vi "RetrieveImage_Main.vi"(8 "error in (no error)":errorcluster, 11 "DevInfo":T1={"Hostname"="", "IPAddress"="", "MAC"="", "SerialNum"="", "Model"="", "Status"="", "FW"="", "OSDesc"="", "ImgTitle"="", "ImgDesc"="", "ImgVer"="", "ImgID"="", "IP Address Request Mode"=1, "SubnetMask"="", "Gateway"="", "DNSServer"=""} {"IP Address Request Mode" items=["Static"=1, "DHCP/Link-Local"=2, "Link-Local Only"=4, "DHCP Only"=8]}) -> (0 "error out":errorcluster)   [LabVIEW 2021]
uses:
  TypeDefs/DevInfo.ctl
  TypeDefs/RetrieveImageStates.ctl
  TypeDefs/AppImageProperties.ctl
  TypeDefs/FPGA_Properties_Element.ctl
  <vilib>/nisyscfg/Software 1.2.ctl
  <vilib>/nisyscfg/Component Type.ctl
  <vilib>/nisyscfg/nisyscfg.lvlib
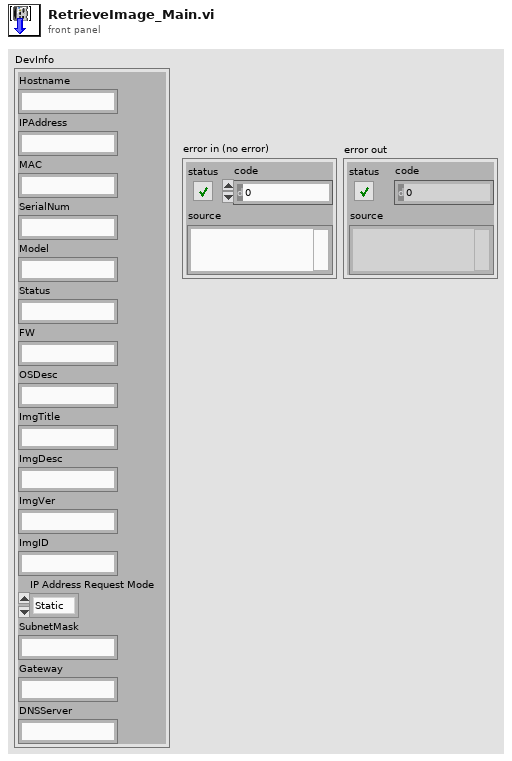
[diagram p1: front panel]
types:
  T1 = typedef "DevInfo.ctl" = cluster{"Hostname":string, "IPAddress":string, "MAC":string, "SerialNum":string, "Model":string, "Status":string, "FW":string, "OSDesc":string, "ImgTitle":string, "ImgDesc":string, "ImgVer":string, "ImgID":string, "IP Address Request Mode":i32, "SubnetMask":string, "Gateway":string, "DNSServer":string}
  T2 = typedef "AppImageProperties.ctl" = cluster{"Name":string, "Version":string, "Time":timestamp, "Description":string, "Key":string, "Chassis":string, "FPGA Properties":T3[], "Model":string, "Retrieve":string[], "Deploy":string[], "Installed Software":string[]}
  T3 = typedef "FPGA_Properties_Element.ctl" = cluster{"Resource Name":string, "Path":path}
  T4 = typedef "RetrieveImageStates.ctl" = enum16{"Get Target Image Info", "Set Image Properties", "Get Installed Software", "Retrieve Image", "Package Image", "Clean Up", "Exit"}
  T5 = cluster{"AppImage Properties":T2, "Image Filepath":path}
  T6 = typedef "nisyscfg.lvlib/Software 1.2.ctl" = cluster{"title":string, "description":string, "ID":string, "version":string, "component type":T7}
  T7 = typedef "nisyscfg.lvlib/Component Type.ctl" = u32
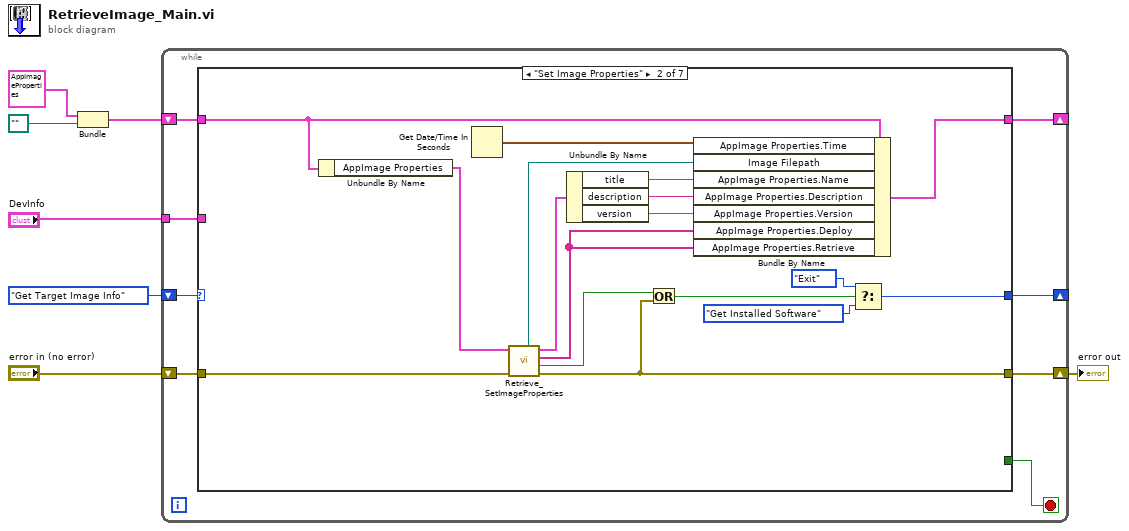
[diagram p0: block diagram]
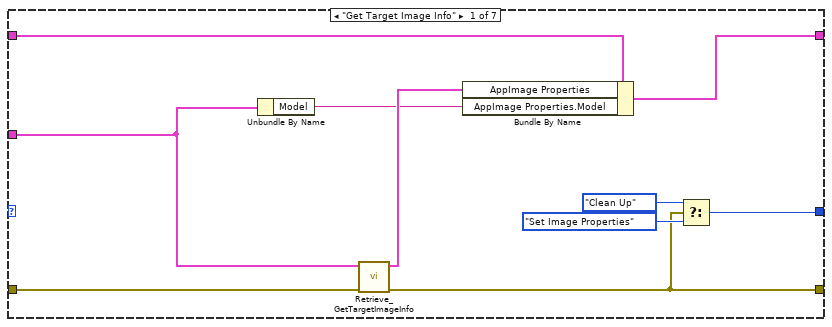
[diagram p2: hidden frame]
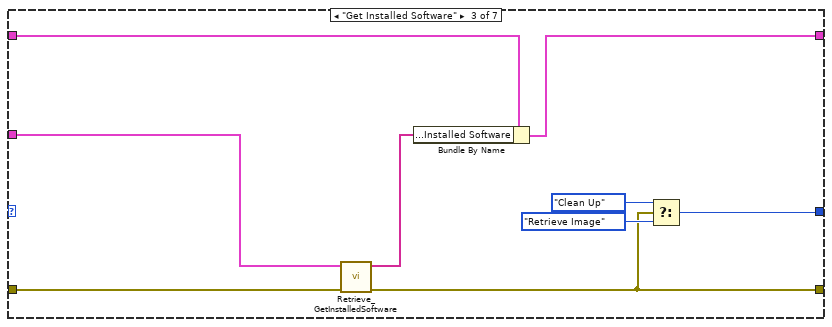
[diagram p3: hidden frame]
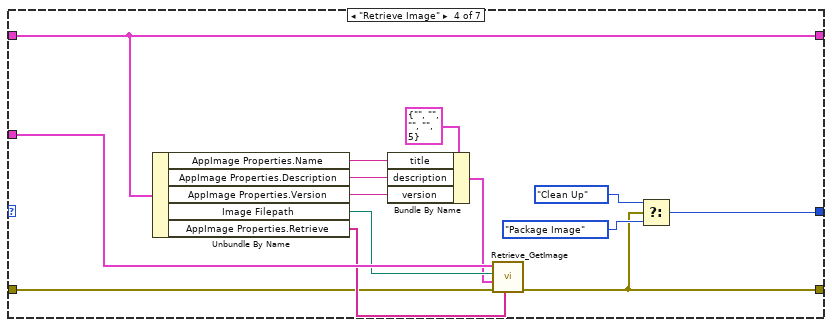
[diagram p4: hidden frame]
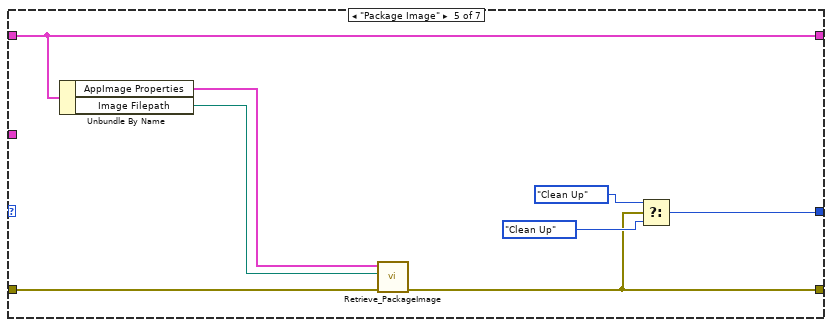
[diagram p5: hidden frame]
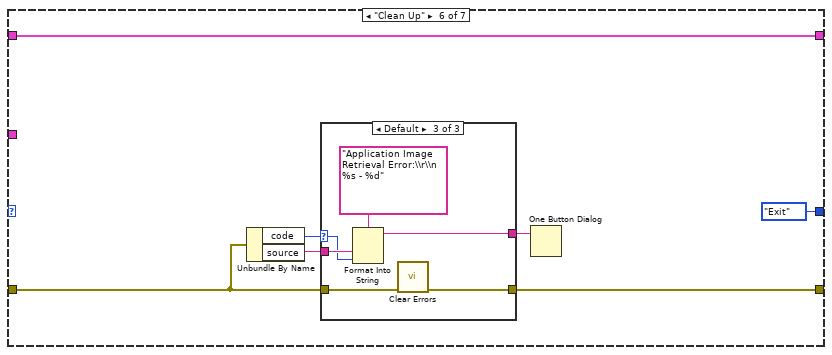
[diagram p6: hidden frame]
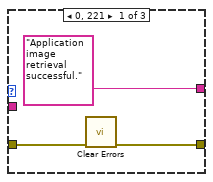
[diagram p7: hidden frame]
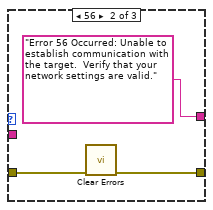
[diagram p8: hidden frame]
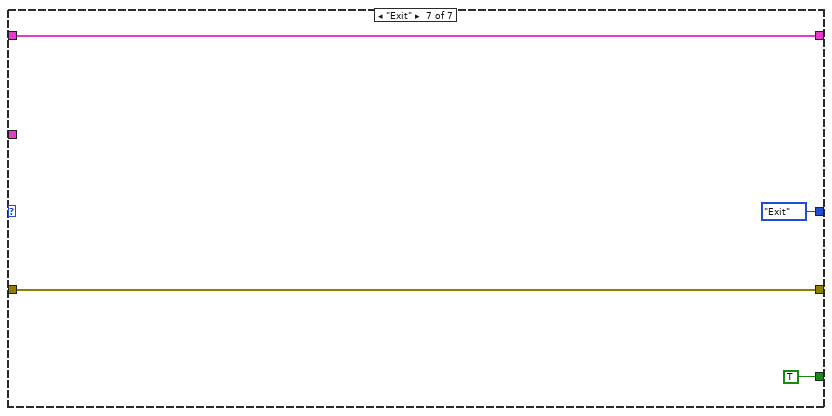
[diagram p9: hidden frame]
diagram:
  n1 = Bundle("AppImage Properties"=T2 {"Name"="", "Version"="", "Time"=timestamp(0 s since 1904-01-01), "Description"="", "Key"="", "Chassis"="", "FPGA Properties"=[], "Model"="", "Retrieve"=[], "Deploy"=[], "Installed Software"=[]}, "Image Filepath"=path "") -> (w5:T5)  [unwired: 1 in]
  n2 = while {
    tunnel: "DevInfo" -> [w12]
    shift-right: [w10] -> _
    shift-left: RetrieveImageStates."Get Target Image Info" -> [w15]
    shift-right: [w11] -> _
    shift-left: w5 -> [w14]
    shift-right: [w9] -> w1
    shift-left: "error in (no error)" -> [w13]
    stop <- w8 stop-if-true
    n3 = case shown="\"Set Image Properties\"" w15 {
      tunnel: w14 -> [w25 w41 w50 w57 w73 w74 w95]
      tunnel: w13 -> [w17 w33 w44 w52 w67 w77 w93]
      tunnel: w12 -> [w22 _ w51 w65 _ _ _]
      tunnel: [w23 w42 w48 w57 w73 w74 w95] -> w11
      tunnel: [w19 w30 w46 w54 w68 RetrieveImageStates."Exit" RetrieveImageStates."Exit"] -> w10
      tunnel: [w16 w29 w43 w53 w66 w76 w93] -> w9
      tunnel: [_ _ _ _ _ _ TRUE] -> w8
      frame "Get Target Image Info" {
        n4 = Unbundle By Name(w22) -> ("Model"=w21:string)
        n5 = call "Retrieve_GetTargetImageInfo.vi"("error in (no error)"=w17, "DevInfo"=w22) -> ("error out"=w16:errorcluster, "AppImage Properties"=w24:T2)  [unwired: 7 in, 1 out]
        n6 = Bundle By Name(cluster=w25, "AppImage Properties"=w24, "AppImage Properties.Model"=w21) -> (w23:T5)
        n7 = Select(t=RetrieveImageStates."Clean Up", s=w16, f=RetrieveImageStates."Set Image Properties") -> (s? t:f=w19:T4)
      }
      frame "Set Image Properties" {
        n8 = Unbundle By Name(w41) -> ("AppImage Properties"=w40:T2)
        n9 = Get Date/Time In Seconds() -> (seconds since 1Jan1904=w26:timestamp)
        n10 = call "Retrieve_SetImageProperties.vi"("error in (no error)"=w33, "AppImage Properties"=w40) -> ("error out"=w29:errorcluster, "Cancelled?"=w28:bool, "Blacklist Out"=w34:string[], "Image Metadata Out"=w38:T6, "Image Filepath"=w39:path)  [unwired: 5 in]
        n11 = Unbundle By Name(w38) -> ("title"=w37:string, "description"=w36:string, "version"=w35:string)
        n12 = Or(x=w28, y=w29) -> (x .or. y?=w27:bool)
        n13 = Bundle By Name(cluster=w41, "AppImage Properties.Time"=w26, "Image Filepath"=w39, "AppImage Properties.Name"=w37, "AppImage Properties.Description"=w36, "AppImage Properties.Version"=w35, "AppImage Properties.Deploy"=w34, "AppImage Properties.Retrieve"=w34) -> (w42:T5)
        n14 = Select(t=RetrieveImageStates."Exit", s=w27, f=RetrieveImageStates."Get Installed Software") -> (s? t:f=w30:T4)
      }
      frame "Get Installed Software" {
        n15 = call "Retrieve_GetInstalledSoftware.vi"("error in (no error)"=w44, "DevInfo"=w51) -> ("error out"=w43:errorcluster, "InstalledSoftware"=w49:string[])  [unwired: 8 in]
        n16 = Bundle By Name(cluster=w50, "AppImage Properties.Installed Software"=w49) -> (w48:T5)
        n17 = Select(t=RetrieveImageStates."Clean Up", s=w43, f=RetrieveImageStates."Retrieve Image") -> (s? t:f=w46:T4)
      }
      frame "Retrieve Image" {
        n18 = Unbundle By Name(w57) -> ("AppImage Properties.Name"=w61:string, "AppImage Properties.Description"=w60:string, "AppImage Properties.Version"=w59:string, "Image Filepath"=w64:path, "AppImage Properties.Retrieve"=w58:string[])
        n19 = Bundle By Name(cluster=T6 {"title"="", "description"="", "ID"="", "version"="", "component type"=5} ("Image Metadata in"), "title"=w61, "description"=w60, "version"=w59) -> (w62:T6)
        n20 = call "Retrieve_GetImage.vi"("File and Directory Blacklist"=w58, "error in (no error)"=w52, "Image Metadata in"=w62, "Image Filepath"=w64, "DevInfo"=w65) -> ("error out"=w53:errorcluster)  [unwired: 6 in]
        n21 = Select(t=RetrieveImageStates."Clean Up", s=w53, f=RetrieveImageStates."Package Image") -> (s? t:f=w54:T4)
      }
      frame "Package Image" {
        n22 = Unbundle By Name(w73) -> ("AppImage Properties"=w72:T2, "Image Filepath"=w71:path)
        n23 = call "Retrieve_PackageImage.vi"("error in (no error)"=w67, "Image Filepath"=w71, "AppImage Properties"=w72) -> ("error out"=w66:errorcluster)  [unwired: 8 in]
        n24 = Select(t=RetrieveImageStates."Clean Up", s=w66, f=RetrieveImageStates."Clean Up") -> (s? t:f=w68:T4)
      }
      frame "Clean Up" {
        n25 = Unbundle By Name(w77) -> ("code"=w79:i32, "source"=w78:string)
        n26 = case shown="Default" w79 {
          selector: w79 -> [_ _ w89]
          tunnel: w78 -> [_ _ w92]
          tunnel: ["Application image retrieval successful." ("source") "Error 56 Occurred: Unable to establish communication with the target.  Verify that your network settings are valid." ("source") w91] -> w80
          tunnel: [w81 w84 w87] -> w76
          tunnel: w77 -> [w82 w85 w88]
          frame 0, 221 {
            n27 = call <vilib>:"Clear Errors.vi"("error in (no error)"=w82) -> ("error out"=w81:errorcluster)  [unwired: 5 in, 1 out]
          }
          frame 56 {
            n28 = call <vilib>:"Clear Errors.vi"("error in (no error)"=w85) -> ("error out"=w84:errorcluster)  [unwired: 5 in, 1 out]
          }
          frame Default {
            n29 = Format Into String(format string="Application Image Retrieval Error:\\r\\n %s - %d", w92, w89) -> (resulting string=w91:string)  [unwired: 2 in, 1 out]
            n30 = call <vilib>:"Clear Errors.vi"("error in (no error)"=w88) -> ("error out"=w87:errorcluster)  [unwired: 5 in, 1 out]
          }
        }
        n31 = One Button Dialog(message=w80) -> ()  [unwired: 2 out]
      }
      frame "Exit" {
      }
    }
  }
  "error out" <- w1
